vi "Test App Broadcast Owned Process Messages.vi"(8 "error in (no error)":errorcluster, 11 "Application Test In":refnum<class "Application Test.lvclass">) -> (0 "error out":errorcluster, 3 "Application Test Out":refnum<class "Application Test.lvclass">)   [LabVIEW 2020, in "Application Test.lvclass"]
uses:
  Application Test.lvclass
  C:/Program Files (x86)/National Instruments/LabVIEW 2020/vi.lib/Asteme/LUnit/Test Case.lvclass
  Mock Process/Mock Process.lvclass
  C:/Users/anton/Documents/GitHub/Triarc-Framework/source/Framework/Process/Process.lvclass
  Framework/Process/Process.lvclass/Process.ctl
  Framework/Application/Application.lvclass/Application.ctl
  <vilib>/Asteme/LUnit/Test Case.lvclass/Test Case.ctl
  <vilib>/Asteme/LUnit/LUnit Assertion Result.lvclass/LUnit Assertion Result.ctl
  Framework/Application/Private/Add Process to Map.vi
  Framework/Application/Private/Start Idle Processes if Running.vi
  Framework/Process/Protected/Messaging/Enqueue Message.vi
  Framework/Process/Public/Lifecycle/Get Lifecycle State.vi
  Framework/Process/Protected/SubVIs/Set Context.vi
  Framework/Process/Private/SubVIs/Wait for finish.vi
  Framework/Process/Private/SubVIs/Set Lifecycle State.vi
  <vilib>/Asteme/LUnit/Palette/Pass.vi
  <vilib>/Asteme/LUnit/Palette/Fail.vi
  <vilib>/Asteme/LUnit/Variant to string.vi
  <vilib>/Asteme/LUnit/Set Assertion Type.vi
  <vilib>/Utility/error.llb/Clear Errors.vi
  Framework/Process/Public/Lifecycle/Leave Process Loop.vi
  <vilib>/Asteme/LUnit/Add test result.vi
  <vilib>/Asteme/LUnit/LUnit Write Passed.vi
  <vilib>/Asteme/LUnit/LUnit Get Test Case.vi
  <vilib>/Asteme/LUnit/Assertion Result/LUnit Get Test Name.vi
  <vilib>/Asteme/LUnit/LUnit Write Message.vi
  <vilib>/Asteme/LUnit/LUnit Write Description.vi
  <vilib>/Asteme/LUnit/LUnit Write Assertion Type.vi
  <vilib>/Asteme/LUnit/Read Test Case Name.vi
  Framework/Application/Application.lvclass
  <vilib>/Utility/error.llb/Error Cluster From Error Code.vi
  Framework/Application/Private/Update Context for Owned Processes.vi
  <vilib>/Utility/Data Type/Get Type Information.vi
  <vilib>/Utility/LVClass/Get LV Class Name.vi
  <vilib>/Asteme/LUnit/LUnit Assertion Result.lvclass
  Framework/Process/Process.lvclass
  <vilib>/Asteme/LUnit/Test Case.lvclass
  Support/Event Helpers/Event Helpers.lvlib
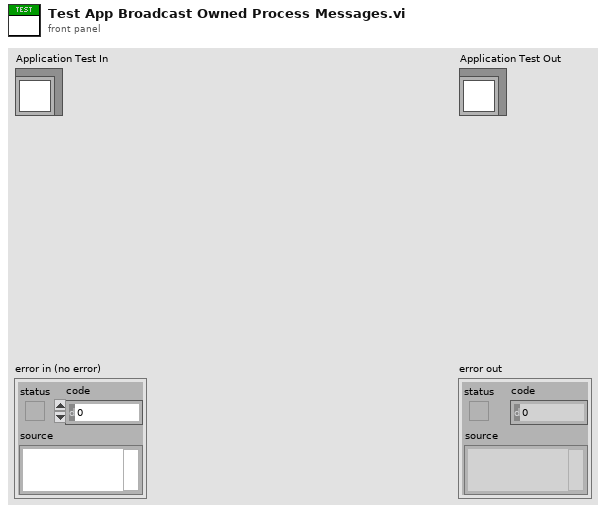
[diagram p1: front panel]
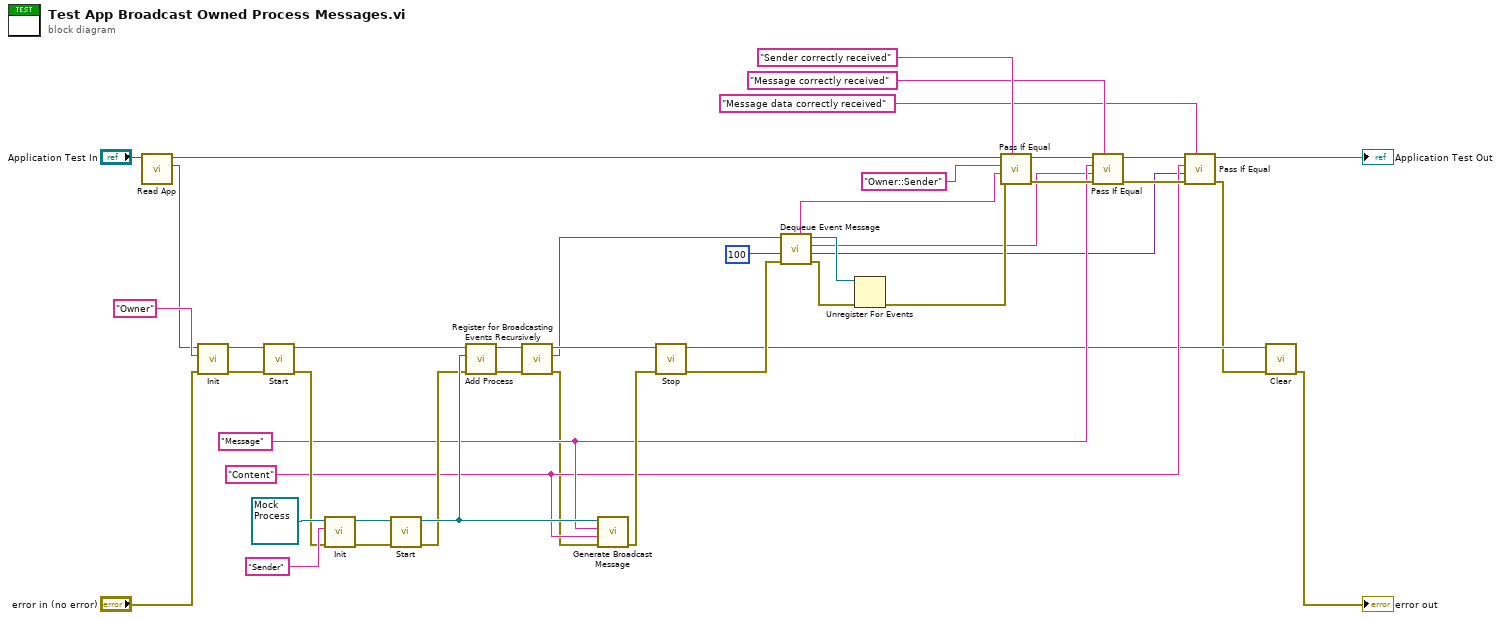
[diagram p0: block diagram]
diagram:
  w13 = "Content" ("Message")
  w14 = "Message" ("Message")
  n1 = call "Read App.vi"("Application Test In"="Application Test In") -> ("App out"=w21:refnum<class "Application.lvclass">, "Application Test Out"=w22:refnum<class "Application Test.lvclass">)  [unwired: 8 in, 1 out]
  n2 = call-dynamic "Init.vi"("error in (no error)"="error in (no error)", "Name"="Owner" ("Message"), "Process In"=w21) -> ("error out"=w42:errorcluster, "Process Out"=w43:refnum<class "Application.lvclass">)  [unwired: 7 in]
  n3 = call "Start.vi"("error in (no error)"=w42, "Process In"=w43) -> ("error out"=w16:errorcluster, "Process Out"=w39:refnum<class "Application.lvclass">)  [unwired: 8 in]
  n4 = call-dynamic "Init.vi"("error in (no error)"=w16, "Name"="Sender" ("Message"), "Mock Process In"=refnum<class "Mock Process.lvclass"> refnum ("Mock Process.lvclass")) -> ("error out"=w25:errorcluster, "Mock Process Out"=w24:refnum<class "Mock Process.lvclass">)  [unwired: 7 in]
  n5 = call "Start.vi"("error in (no error)"=w25, "Process In"=w24) -> ("error out"=w15:errorcluster, "Process Out"=w20:refnum<class "Mock Process.lvclass">)  [unwired: 8 in]
  n6 = call "Add Process.vi"("error in (no error)"=w15, "Process"=w20, "Rig In"=w39) -> ("error out"=w7:errorcluster, "Rig Out"=w8:refnum<class "Application.lvclass">)  [unwired: 7 in]
  n7 = call "Register for Broadcasting Events Recursively.vi"("error in (no error)"=w7, "Application In"=w8) -> ("error out"=w5:errorcluster, "Event Registration Refnum Out"=w4:refnum<event-registration>, "Application Out"=w6:refnum<class "Application.lvclass">)  [unwired: 7 in]
  n8 = call "Generate Broadcast Message.vi"("error in (no error)"=w5, "Message Data"=w13, "Message"=w14, "Mock Process In"=w20) -> ("error out"=w18:errorcluster)  [unwired: 6 in, 1 out]
  n9 = call "Stop.vi"("error in (no error)"=w18, "Process In"=w6) -> ("error out"=w41:errorcluster, "Process Out"=w3:refnum<class "Application.lvclass">)  [unwired: 7 in, 1 out]
  n10 = call "Dequeue Event Message.vi"("error in (no error)"=w41, "Timeout (-1)"=100, "Event Registration Refnum"=w4) -> ("error out"=w9:errorcluster, "Message Data"=w11:variant, "Message"=w12:string, "Event Registration Refnum Out"=w38:refnum<event-registration>, "Sender"=w37:string)  [unwired: 3 in, 1 out]
  n11 = Unregister For Events(event registration refnum=w38, error in=w9) -> (error out=w31:errorcluster)
  n12 = call <vilib>:"Pass If Equal.vi"("Description"="Sender correctly received", "error in (no error)"=w31, "Actual"=w37, "Expected"="Owner::Sender" ("Message"), "Test Case In"=w22) -> ("error out"=w34:errorcluster, "Test Case Out"=w35:refnum<class "Application Test.lvclass">)  [unwired: 5 in]
  n13 = call <vilib>:"Pass If Equal.vi"("Description"="Message correctly received", "error in (no error)"=w34, "Actual"=w12, "Expected"=w14, "Test Case In"=w35) -> ("error out"=w32:errorcluster, "Test Case Out"=w33:refnum<class "Application Test.lvclass">)  [unwired: 5 in]
  n14 = call <vilib>:"Pass If Equal.vi"("Description"="Message data correctly received", "error in (no error)"=w32, "Actual"=w11, "Expected"=w13, "Test Case In"=w33) -> ("error out"=w2:errorcluster, "Test Case Out"=→"Application Test Out":refnum<class "Application Test.lvclass">)  [unwired: 5 in]
  n15 = call-dynamic "Clear.vi"("error in (no error)"=w2, "Application In"=w3) -> ("error out"=→"error out":errorcluster)  [unwired: 9 in]
